vi "C4If_getInterfaceName.vi"(0 "c4if in":refnum<k24>, 11 "error in (no error)":errorcluster) -> (4 "c4if out":refnum<k24>, 6 "interface name out":string, 15 "error out":errorcluster)   [LabVIEW 2015, in "libC4HdlLV.lvlib"]
uses:
  libC4HdlLV.lvlib
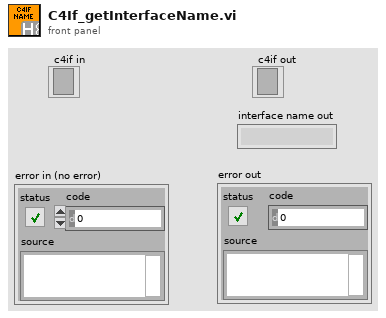
[diagram p1: front panel]
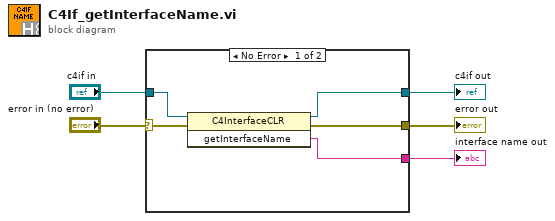
[diagram p0: block diagram]
diagram:
  n1 = case shown="No Error" "error in (no error)" {
    selector: "error in (no error)" -> [w10 w12]
    tunnel: [w8 w12] -> w5
    tunnel: [w7 _] -> w1
    tunnel: "c4if in" -> [w9 w11]
    tunnel: [w6 w11] -> w2
    frame No Error {
      n2 = invoke class="C4InterfaceCLR" method="getInterfaceName"(reference=w9, error in=w10) -> (reference out=w6:refnum<k24>, error out=w8:errorcluster, "getInterfaceName"=w7:string)  [unwired: 1 in]
    }
    frame Error {
    }
  }
  "error out" <- w5
  "c4if out" <- w2
  "interface name out" <- w1
